vi "Main.vi"(11 "Module Admin":refnum<class "Delacor_lib_QMH_Module Admin.lvclass">) -> ()   [LabVIEW 2020, in "UI.lvlib"]
doc: "This template is based off of the Queued Message Handler design pattern and the Queued Message Handler project template that ships with LabVIEW.\n\nThe main difference is that the queue is private to this module and communication between modules is performed via Broadcast and Request events.\n\nRequest events are wrapped in public API methods and are handled in the Event Handling Loop (EHL) of this VI. Any module can register for Broadcast events sent by this module. The EHL generates messages based on user interface actions.\n\nThe Message Handling Loop (MHL) processes messages generated by the EHL, or by other messages. The messages are string values, so new messages can be added easily to the Message Cases case structure in the MHL. Each message cluster can also provide an optional value for Message Data, which is a variant that can be converted to whatever message-specific data is required.\n_____\nBased on DQMH Project Template 6.0.0.91."
uses:
  UI.lvlib
  <vilib>/Delacor/Delacor QMH/Libraries/Module Admin_class/Delacor_lib_QMH_Module Admin.lvclass
  Module Data--cluster.ctl
  Stop Argument--cluster.ctl
  <vilib>/Delacor/Delacor QMH/Libraries/Message Queue_class/Delacor_lib_QMH_Message Queue.lvclass/Delacor_lib_QMH_Message Queue.ctl
  <vilib>/Delacor/Delacor QMH/Libraries/Module Admin_class/Delacor_lib_QMH_Module Admin.lvclass/Delacor_lib_QMH_Module Admin.ctl
  <vilib>/Utility/miscctls.llb/LVPointTypeDef.ctl
  <vilib>/Delacor/Delacor QMH/Libraries/Message Queue_class/Delacor_lib_QMH_Enqueue Message (Single).vi
  <vilib>/Delacor/Delacor QMH/Libraries/Module Admin_class/Delacor_lib_QMH_Get External Launch.vi
  <vilib>/Utility/error.llb/Error Cluster From Error Code.vi
  <vilib>/ErrorRing/Error Ring.xnode
  <vilib>/Delacor/Delacor QMH/Libraries/Message Queue_class/Delacor_lib_QMH_Message Queue.lvclass
  Dinero/Dinero.lvlib
  Manejador Turnos/Manejador Turnos.lvlib
  Paquetes Disponibles/Paquetes Disponibles.lvlib
  Contabilidad/Contabilidad.lvlib
panel:
  in  "PARO TOTAL":bool
  in  "PARO":bool
  in  "Contabilidad":bool
  out "Status":string
  out "error out":errorcluster
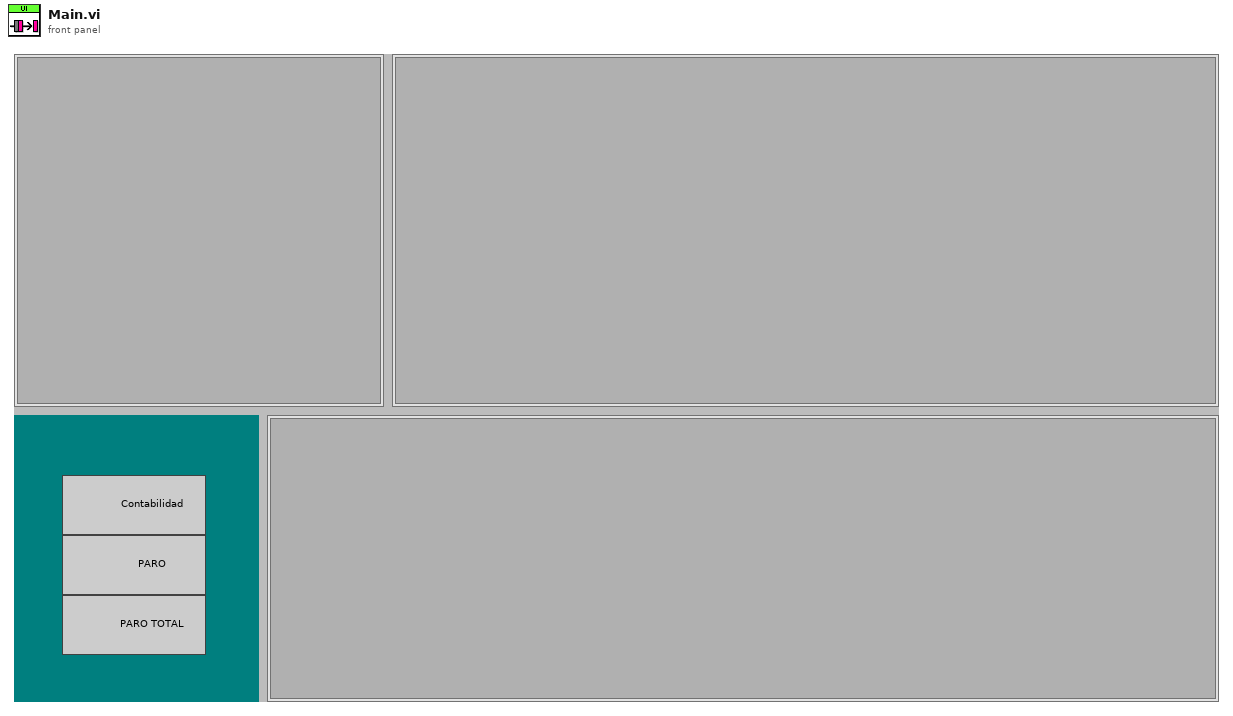
[diagram p1: front panel]
types:
  T1 = typedef "UI.lvlib/Request Events--cluster.ctl" = cluster{"Stop Module":refnum<user-event>, "Show Panel":refnum<user-event>, "Hide Panel":refnum<user-event>, "Get Module Execution Status":refnum<user-event>, "Show Diagram":refnum<user-event>, "Actualizar Cambio":refnum<user-event>, "Credito 0":refnum<user-event>}
  T2 = typedef "Contabilidad.lvlib/Broadcast Events--cluster.ctl" = cluster{"Module Did Init":refnum<user-event>, "Status Updated":refnum<user-event>, "Error Reported":refnum<user-event>, "Module Did Stop":refnum<user-event>, "Update Module Execution Status":refnum<user-event>}
  T3 = typedef "Manejador Turnos.lvlib/Broadcast Events--cluster.ctl" = cluster{"Module Did Init":refnum<user-event>, "Status Updated":refnum<user-event>, "Error Reported":refnum<user-event>, "Module Did Stop":refnum<user-event>, "Update Module Execution Status":refnum<user-event>}
  T4 = typedef "Paquetes Disponibles.lvlib/Broadcast Events--cluster.ctl" = cluster{"Module Did Init":refnum<user-event>, "Status Updated":refnum<user-event>, "Error Reported":refnum<user-event>, "Module Did Stop":refnum<user-event>, "Update Module Execution Status":refnum<user-event>, "Servicio Seleccionado":refnum<user-event>, "Actualizar Credito":refnum<user-event>, "Actualizar Cambio":refnum<user-event>}
  T5 = typedef "Dinero.lvlib/Broadcast Events--cluster.ctl" = cluster{"Module Did Init":refnum<user-event>, "Status Updated":refnum<user-event>, "Error Reported":refnum<user-event>, "Module Did Stop":refnum<user-event>, "Update Module Execution Status":refnum<user-event>, "Credito":refnum<user-event>}
  T6 = typedef "UI.lvlib/Module Data--cluster.ctl" = cluster{"Status":string}
  T7 = enum32{"invalid lock state", "Not Locked", "Locked (No Password)", "Password-protected"}
  T8 = typedef "UI.lvlib/Stop Argument--cluster.ctl" = cluster{"Origin":string, "Exit via Stop Module Req?":bool, "Wait for Module to stop?":bool}
  T9 = enum32{"Invalid", "Standard", "Closed", "Hidden", "Minimized", "Maximized"}
  T10 = typedef "LVPointTypeDef.ctl" = cluster{"Horizontal":i16, "Vertical":i16}
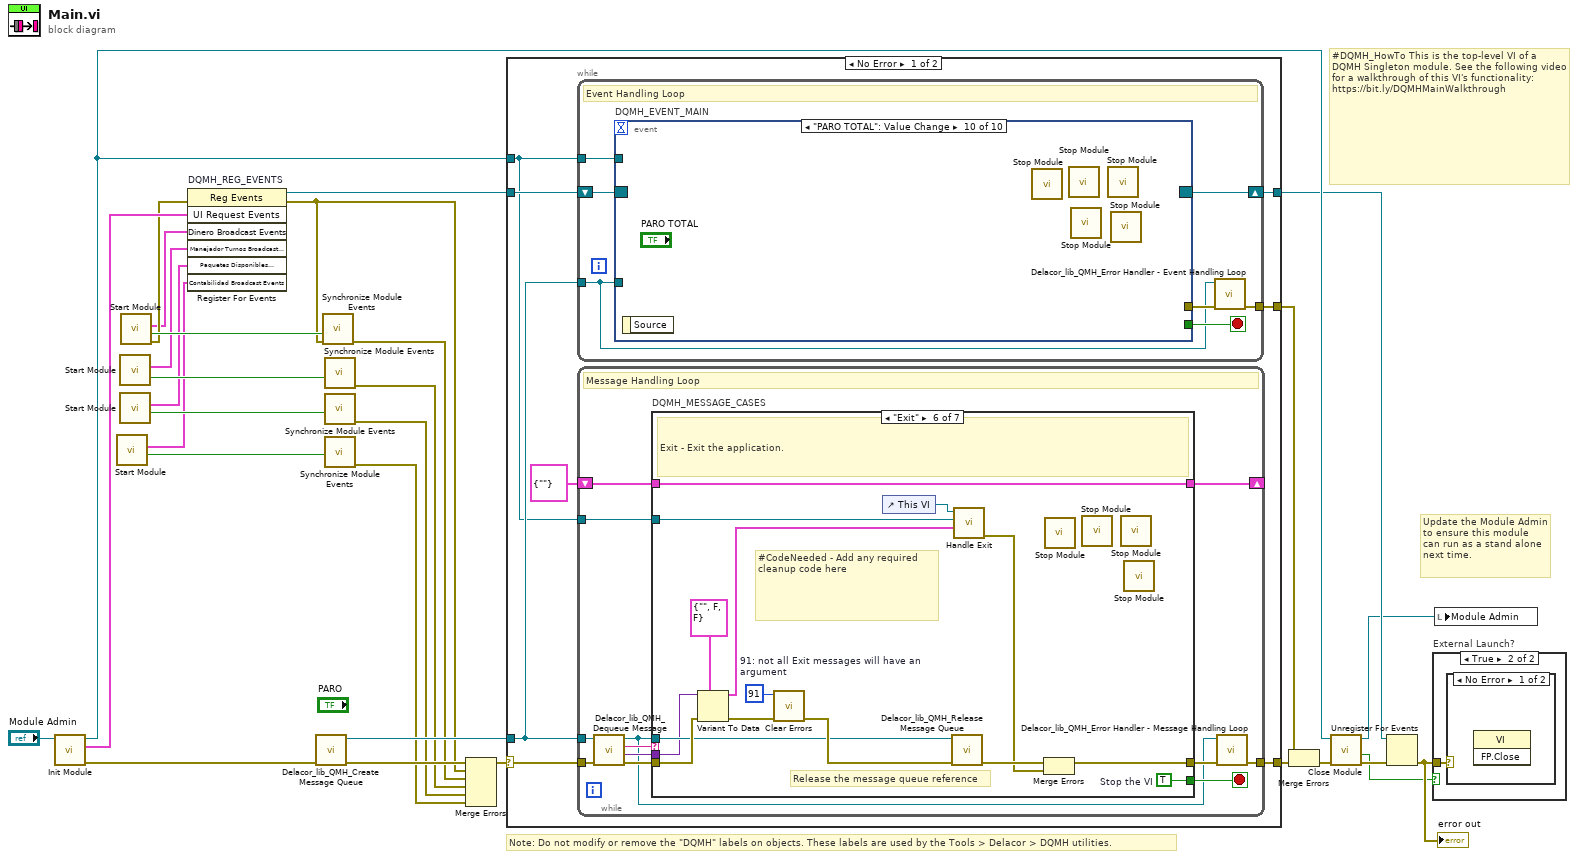
[diagram p0: block diagram]
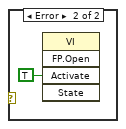
[diagram p3: hidden frame]
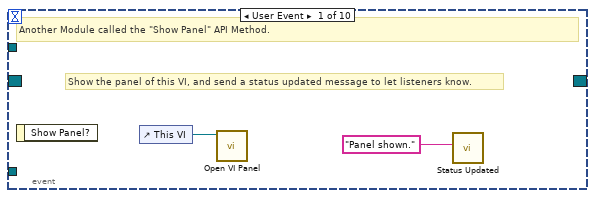
[diagram p4: hidden frame]
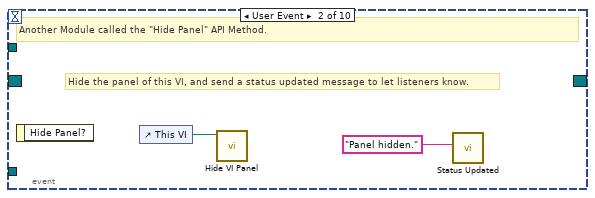
[diagram p5: hidden frame]
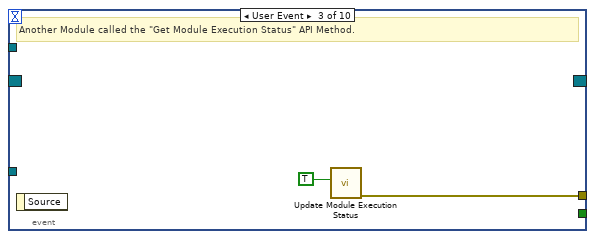
[diagram p6: hidden frame]
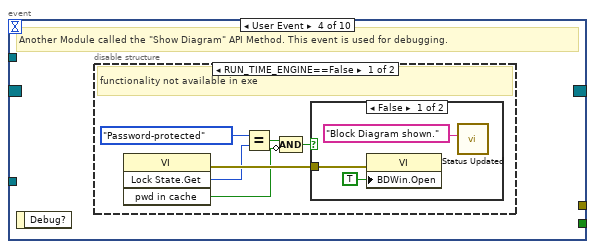
[diagram p7: hidden frame]
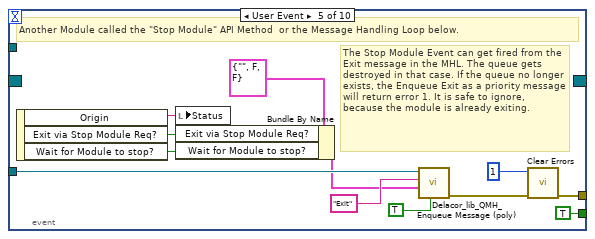
[diagram p10: hidden frame]
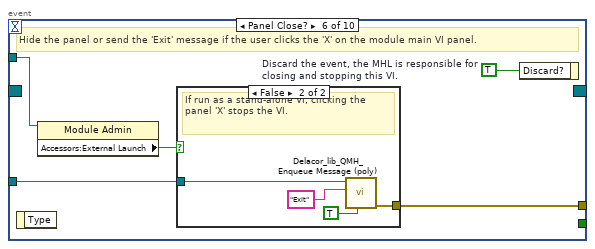
[diagram p11: hidden frame]
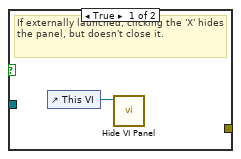
[diagram p12: hidden frame]
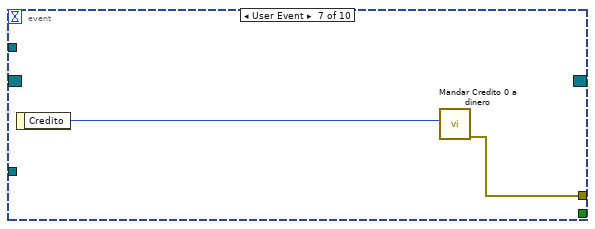
[diagram p13: hidden frame]
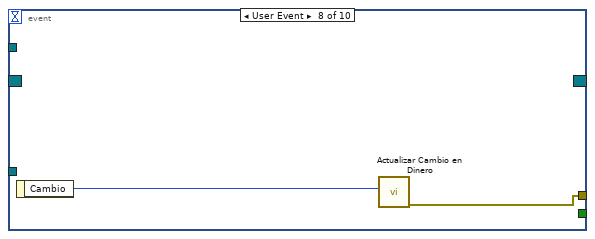
[diagram p14: hidden frame]
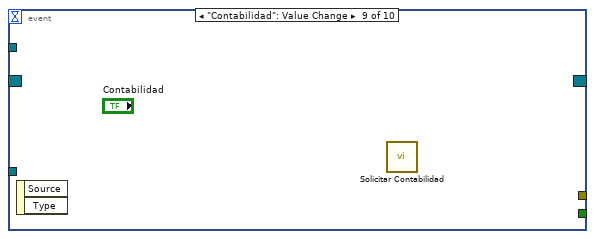
[diagram p15: hidden frame]
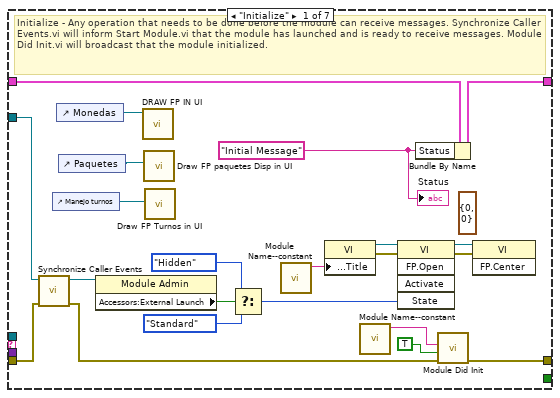
[diagram p16: hidden frame]
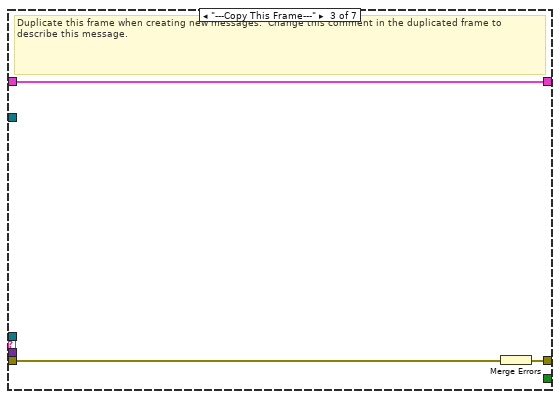
[diagram p18: hidden frame]
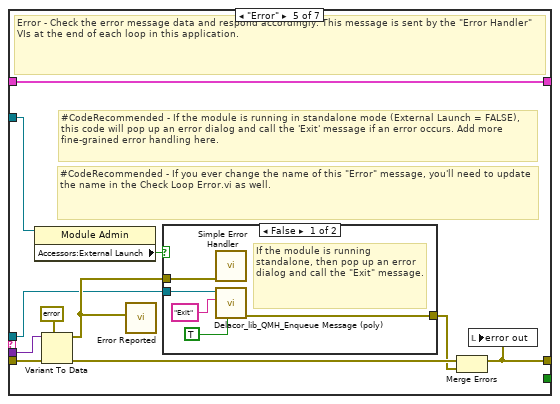
[diagram p20: hidden frame]
diagram:
  # "#DQMH_HowTo This is the top-level VI of a DQMH Singleton module. See the following video for a walkthrough of this VI's functionality: https://bit.ly/DQMHMainWalkthrough"
  # "Note: Do not modify or remove the \"DQMH\" labels on objects. These labels are used by the Tools > Delacor > DQMH utilities."
  # "Update the Module Admin to ensure this module can run as a stand alone next time."
  n1 = call "Init Module.vi"("Singleton Module Admin in"="Module Admin") -> ("error out"=w29:errorcluster, "UI Request Events"=w19:T1, "Singleton Module Admin out"=w22:refnum<class "Delacor_lib_QMH_Module Admin.lvclass">)  [unwired: 8 in]
  n2 = call "Start Module.vi"() -> ("Wait for Event Sync?"=w3:bool, "Contabilidad Broadcast Events"=w2:T2)  [unwired: 8 in, 2 out]
  n3 = call "Start Module.vi"() -> ("Wait for Event Sync?"=w9:bool, "Manejador Turnos Broadcast Events"=w5:T3)  [unwired: 8 in, 2 out]
  n4 = call "Start Module.vi"() -> ("Wait for Event Sync?"=w8:bool, "Paquetes Disponibles Broadcast Events"=w4:T4)  [unwired: 8 in, 2 out]
  n5 = call "Start Module.vi"() -> ("error out"=w13:errorcluster, "Wait for Event Sync?"=w14:bool, "Dinero Broadcast Events"=w10:T5)  [unwired: 8 in, 1 out]
  n6 = register-events "DQMH_REG_EVENTS"(error in=w13, w19, w10, w5, w4, w2) -> (reference out=w20:refnum<event-registration>, error out=w12:errorcluster)  [unwired: 1 in]
  n7 = call <vilib>:"Delacor_lib_QMH_Create Message Queue.vi"("error in"=w29) -> ("error out"=w24:errorcluster, "Message Queue"=w18:refnum<class "Delacor_lib_QMH_Message Queue.lvclass">)  [unwired: 9 in]
  n8 = call "Synchronize Module Events.vi"("error in"=w12, "Wait for Event Sync?"=w14) -> ("error out"=w11:errorcluster)  [unwired: 9 in]
  n9 = call "Synchronize Module Events.vi"("Wait for Event Sync?"=w9) -> ("error out"=w7:errorcluster)  [unwired: 10 in]
  n10 = call "Synchronize Module Events.vi"("Wait for Event Sync?"=w8) -> ("error out"=w6:errorcluster)  [unwired: 10 in]
  n11 = call "Synchronize Module Events.vi"("Wait for Event Sync?"=w3) -> ("error out"=w1:errorcluster)  [unwired: 10 in]
  n12 = Merge Errors(w24, w12, w11, w7, w6, w1) -> (w23:errorcluster)
  n13 = case shown="No Error" w23 {
    selector: w23 -> [w36 w175]
    tunnel: [w38 w174] -> w30
    tunnel: [w35 w180] -> w21
    tunnel: w20 -> [w33 w180]
    tunnel: w18 -> [w32 w173]
    tunnel: [w37 _] -> w27
    tunnel: w22 -> [w31 w176]
    frame No Error {
      n14 = while {
        tunnel: w32 -> [w39]
        shift-right: [w42] -> w35
        shift-left: w33 -> [w43]
        tunnel: [w44] -> w37
        tunnel: w31 -> [w40]
        stop <- w41 stop-if-true
        # "Event Handling Loop"
        n15 = event "DQMH_EVENT_MAIN" shown="[9] \"PARO TOTAL\": Value Change" {
          selector: w43 -> [_ _ _ _ _ _ _ _ _ _]
          dyn-events: [_ _ _ _ _ _ _ _ _ _] -> w42
          timeout: _ -> [_ _ _ _ _ _ _ _ _ _]
          tunnel: [_ _ _ _ TRUE ("Discard?") _ _ _ _ _] -> w41
          tunnel: w39 -> [_ _ _ _ w68 w75 _ _ _ _]
          tunnel: [_ _ w51 _ w71 w77 w83 w86 _ _] -> w45
          tunnel: w40 -> [_ _ _ _ _ w74 _ _ _ _]
          event User Event {
            # "Show the panel of this VI, and send a status updated message to let listeners know."
            # "Another Module called the \"Show Panel\" API Method."
            n16 = event-data() -> ()  [unwired: 1 in, 1 out]
            n17 = control-ref of="This VI"() -> (w47:refnum<vi>)
            n18 = call "Open VI Panel.vi"("VI"=w47) -> ()  [unwired: 10 in, 1 out]
            n19 = call "Status Updated.vi"("Status"="Panel shown." ("format string")) -> ()  [unwired: 10 in, 1 out]
          }
          event User Event {
            # "Hide the panel of this VI, and send a status updated message to let listeners know."
            # "Another Module called the \"Hide Panel\" API Method."
            n20 = event-data() -> ()  [unwired: 1 in, 1 out]
            n21 = control-ref of="This VI"() -> (w49:refnum<vi>)
            n22 = call "Hide VI Panel.vi"("VI"=w49) -> ()  [unwired: 10 in, 1 out]
            n23 = call "Status Updated.vi"("Status"="Panel hidden." ("format string")) -> ()  [unwired: 10 in, 1 out]
          }
          event User Event {
            # "Another Module called the \"Get Module Execution Status\" API Method."
            n24 = event-data() -> ()  [unwired: 1 in, 1 out]
            n25 = call "Update Module Execution Status.vi"("Running?"=TRUE) -> ("error out"=w51:errorcluster)  [unwired: 10 in]
          }
          event User Event {
            # "Another Module called the \"Show Diagram\" API Method. This event is used for debugging."
            n26 = event-data() -> ()  [unwired: 1 in, 1 out]
            n27 = disable-structure shown="RUN_TIME_ENGINE==False" {
              frame condition #0 (active) {
                # "functionality not available in exe"
                n28 = invoke class="VI" method="Lock State.Get"() -> (error out=w57:errorcluster, "Get Lock State"=w56:T7, "pwd in cache"=w53:bool)  [unwired: 4 in, 1 out]
                n29 = Equal?(x=T7."Password-protected", y=w56) -> (x = y?=w54:bool)
                n30 = Compound Arithmetic op=AND(w54, invert w53) -> (w52:bool)
                n31 = case shown="False" w52 {
                  tunnel: w57 -> [w60 _]
                  frame False {
                    n32 = property class="VI"(error in=w60, "BDWin.Open"=TRUE ("Block Diagram Window:Open")) -> ()  [unwired: 1 in, 2 out]
                    n33 = call "Status Updated.vi"("Status"="Block Diagram shown." ("format string")) -> ()  [unwired: 10 in, 1 out]
                  }
                  frame True {
                    # "Password-protected VI, and the password is not in the cache. Do not show the diagram."
                  }
                }
              }
              frame condition #1 {
              }
            }
          }
          event User Event {
            # "The Stop Module Event can get fired from the Exit message in the MHL. The queue gets destroyed in that case. If the queue no longer exists, the Enqueue Exit as a priority message will return error 1. It is safe to ignore, because the module is already exiting."
            # "Another Module called the \"Stop Module\" API Method  or the Message Handling Loop below."
            n34 = event-data() -> ("Origin"=w67:string, "Exit via Stop Module Req?"=w63:bool, "Wait for Module to stop?"=w62:bool)  [unwired: 1 in]
            n35 = local write "Status"(w67) -> ()
            n36 = Bundle By Name(cluster=T8 {"Origin"="", "Exit via Stop Module Req?"=FALSE, "Wait for Module to stop?"=FALSE} ("Stop Argument"), "Exit via Stop Module Req?"=w63, "Wait for Module to stop?"=w62) -> (w61:T8)
            n37 = call-poly <vilib>:"Delacor_lib_QMH_Enqueue Message (poly).vi"("Priority Message? (F)"=TRUE, "Message Data"=w61, "Message"="Exit", "Message Queue in"=w68) -> ("error out"=w72:errorcluster)  [unwired: 6 in, 1 out]
            n38 = call <vilib>:"Clear Errors.vi"("error in (no error)"=w72, "specific error code to clear (0: all)"=1) -> ("error out"=w71:errorcluster)  [unwired: 4 in, 1 out]
          }
          event Panel Close? {
            w76 = TRUE  # Discard the event, the MHL is responsible for closing and stopping this VI.
            # "Hide the panel or send the 'Exit' message if the user clicks the 'X' on the module main VI panel."
            n39 = event-data() -> ()  [unwired: 1 in, 1 out]
            n40 = property class="Module Admin"(reference=w74) -> ("Accessors:External Launch"=w73:bool)  [unwired: 1 in, 2 out]
            n41 = case shown="False" w73 {
              tunnel: w75 -> [_ w81]
              tunnel: [_ w82] -> w77
              frame True {
                # "If externally launched, clicking the 'X' hides the panel, but doesn't close it."
                n42 = control-ref of="This VI"() -> (w78:refnum<vi>)
                n43 = call "Hide VI Panel.vi"("VI"=w78) -> ()  [unwired: 10 in, 1 out]
              }
              frame False {
                # "If run as a stand-alone VI, clicking the panel 'X' stops the VI."
                n44 = call-poly <vilib>:"Delacor_lib_QMH_Enqueue Message (poly).vi"("Priority Message? (F)"=TRUE, "Message"="Exit", "Message Queue in"=w81) -> ("error out"=w82:errorcluster)  [unwired: 7 in, 1 out]
              }
            }
            n45 = event-data("Discard?"=w76) -> ()  [unwired: 1 in, 1 out]
          }
          event User Event {
            n46 = event-data() -> ("Credito"=w84:i32)  [unwired: 1 in]
            n47 = call "Mandar Credito 0 a dinero.vi"("Credito"=w84) -> ("error out"=w83:errorcluster)  [unwired: 10 in]
          }
          event User Event {
            n48 = event-data() -> ("Cambio"=w85:i32)  [unwired: 1 in]
            n49 = call "Actualizar Cambio en Dinero.vi"("Cambio"=w85) -> ("error out"=w86:errorcluster)  [unwired: 10 in]
          }
          event "Contabilidad": Value Change {
            n50 = event-data() -> ()  [unwired: 1 in, 2 out]
            n51 = call "Solicitar Contabilidad.vi"() -> ()  [unwired: 12 in]
          }
          event "PARO TOTAL": Value Change {
            n52 = event-data() -> ()  [unwired: 1 in, 1 out]
            n53 = call "Stop Module.vi"() -> ()  [unwired: 11 in, 1 out]
            n54 = call "Stop Module.vi"() -> ()  [unwired: 11 in, 1 out]
            n55 = call "Stop Module.vi"() -> ()  [unwired: 11 in, 1 out]
            n56 = call "Stop Module.vi"() -> ()  [unwired: 11 in, 1 out]
            n57 = call "Stop Module.vi"() -> ()  [unwired: 11 in, 1 out]
          }
        }
        n58 = call-dynamic "Delacor_lib_QMH_Error Handler - Event Handling Loop.vi"("error in"=w45, "Message Queue in"=w39) -> ("dup error in"=w44:errorcluster)  [unwired: 8 in, 1 out]
      }
      n59 = while {
        tunnel: w32 -> [w89]
        shift-right: [w93] -> _
        shift-left: T6 {"Status"=""} ("Data Cluster") -> [w94]
        tunnel: w36 -> [w97]
        tunnel: [w95] -> w38
        tunnel: w31 -> [w87]
        stop <- w92 stop-if-true
        # "Message Handling Loop"
        n60 = call-dynamic "Delacor_lib_QMH_Dequeue Message.vi"("error in"=w97, "Message Queue in"=w89) -> ("error out"=w96:errorcluster, "Message Data"=w90:variant, "Message"=w91:string, "Message Queue out"=w88:refnum<class "Delacor_lib_QMH_Message Queue.lvclass">)  [unwired: 6 in]
        n61 = case "DQMH_MESSAGE_CASES" shown="\"Exit\"" w91 {
          selector: w91 -> [_ _ _ _ _ _ w160]
          tunnel: w88 -> [_ _ _ _ w130 w152 _]
          tunnel: w96 -> [w118 w122 w125 w127 w137 w158 w162]
          tunnel: [w116 w122 w124 w127 w133 w155 w163] -> w98
          tunnel: w94 -> [w107 w121 w123 w126 w132 w151 w161]
          tunnel: [w106 w121 w123 w126 w132 w151 w161] -> w93
          tunnel: [_ _ _ _ _ w150 _] -> w92
          tunnel: w90 -> [_ _ _ _ w131 w149 _]
          tunnel: w87 -> [w108 _ _ _ w129 w144 _]
          frame "Initialize" {
            (unwired) T10 {"Horizontal"=0, "Vertical"=0} ("Origin")
            w102 = "Initial Message" ("Initial Message")
            # "Initialize - Any operation that needs to be done before the module can receive messages. Synchronize Caller Events.vi will inform Start Module.vi that the module has launched and is ready to receive messages. Module Did Init.vi will broadcast that the module initialized."
            n62 = call "Synchronize Caller Events.vi"("error in (no error)"=w118, "Singleton Module Admin in"=w108) -> ("error out"=w117:errorcluster, "Singleton Module Admin out"=w103:refnum<class "Delacor_lib_QMH_Module Admin.lvclass">)  [unwired: 8 in]
            n63 = control-ref of="Manejo turnos"() -> (w99:refnum<vi>)
            n64 = control-ref of="Monedas"() -> (w101:refnum<vi>)
            n65 = control-ref of="Paquetes"() -> (w100:refnum<vi>)
            n66 = property class="Module Admin"(reference=w103) -> ("Accessors:External Launch"=w112:bool)  [unwired: 1 in, 2 out]
            n67 = call "DRAW FP IN UI.vi"("Sub Panel Dinero"=w101) -> ()  [unwired: 10 in, 1 out]
            n68 = call "Draw FP paquetes Disp in UI.vi"("Sub Panel Paquetes"=w100) -> ()  [unwired: 10 in, 1 out]
            n69 = call "Draw FP Turnos in UI.vi"("Sub Panel Trunos"=w99) -> ()  [unwired: 10 in, 1 out]
            n70 = Select(t=T9."Hidden" ("State"), s=w112, f=T9."Standard" ("State")) -> (s? t:f=w109:T9)
            n71 = call "Module Name--constant.vi"() -> ("Module Name"=w115:string)  [unwired: 11 in]
            n72 = property class="VI"("Front Panel.Title"=w115) -> (reference out=w114:refnum<vi>, error out=w120:errorcluster)  [unwired: 2 in]
            n73 = call "Module Name--constant.vi"() -> ("Module Name"=w104:string)  [unwired: 11 in]
            n74 = invoke class="VI" method="FP.Open"(reference=w114, error in=w120, "State"=w109) -> (reference out=w113:refnum<vi>, error out=w119:errorcluster)  [unwired: 2 in, 3 out]
            n75 = Bundle By Name(cluster=w107, "Status"=w102) -> (w106:T6)
            n76 = call "Module Did Init.vi"("error in (no error)"=w117, "Initialized?"=TRUE, "Origin"=w104) -> ("error out"=w116:errorcluster)  [unwired: 8 in]
            n77 = invoke class="VI" method="FP.Center"(reference=w113, error in=w119) -> ()  [unwired: 1 in, 3 out]
            "Status" <- w102
          }
          frame "---Module Specific---" {
            # "Separator -- The following cases handle messages specific to this Module."
          }
          frame "---Copy This Frame---" {
            # "Duplicate this frame when creating new messages.  Change this comment in the duplicated frame to describe this message."
            n78 = Merge Errors(w125) -> (w124:errorcluster)
          }
          frame "---Exit and Error Handling---" {
            # "Separator - The following cases handle errors and exit messages."
          }
          frame "Error" {
            # "#CodeRecommended - If you ever change the name of this \"Error\" message, you'll need to update the name in the Check Loop Error.vi as well."
            # "#CodeRecommended - If the module is running in standalone mode (External Launch = FALSE), this code will pop up an error dialog and call the 'Exit' message if an error occurs. Add more fine-grained error handling here."
            # "Error - Check the error message data and respond accordingly. This message is sent by the \"Error Handler\" VIs at the end of each loop in this application."
            n79 = property class="Module Admin"(reference=w129) -> ("Accessors:External Launch"=w128:bool)  [unwired: 1 in, 2 out]
            n80 = Variant To Data(error in=w137, type=errorcluster {"status"=FALSE, "code"=0, "source"=""} ("error constant"), Variant=w131) -> (data=w138:errorcluster, error out=w135:errorcluster)
            n81 = call "Error Reported.vi"("Error"=w138) -> ()  [unwired: 10 in, 1 out]
            n82 = case shown="False" w128 {
              tunnel: [w143 _] -> w134
              tunnel: w130 -> [w141 _]
              tunnel: w138 -> [w142 _]
              frame False {
                # "If the module is running standalone, then pop up an error dialog and call the \"Exit\" message."
                n83 = call <vilib>:"Simple Error Handler.vi"("error in (no error)"=w142) -> ()  [unwired: 4 in, 5 out]
                n84 = call-poly <vilib>:"Delacor_lib_QMH_Enqueue Message (poly).vi"("Priority Message? (F)"=TRUE, "Message"="Exit", "Message Queue in"=w141) -> ("error out"=w143:errorcluster)  [unwired: 7 in, 1 out]
              }
              frame True {
                # "If the module was launched externally, calling the Error Reported broadcast VI is the only action performed by the \"Error\" message. The module's caller can then process the error appropriately."
              }
            }
            n85 = Merge Errors(w135, w134) -> (w133:errorcluster)
            n86 = local write "error out"(w133) -> ()
          }
          frame "Exit" {
            w148 = 91  # 91: not all Exit messages will have an argument
            w150 = TRUE  # Stop the VI
            # "Release the message queue reference"
            # "#CodeNeeded - Add any required cleanup code here"
            # "Exit - Exit the application."
            n87 = Variant To Data(error in=w158, type=T8 {"Origin"="", "Exit via Stop Module Req?"=FALSE, "Wait for Module to stop?"=FALSE} ("Stop Argument"), Variant=w149) -> (data=w146:T8, error out=w154:errorcluster)
            n88 = call <vilib>:"Clear Errors.vi"("error in (no error)"=w154, "specific error code to clear (0: all)"=w148) -> ("error out"=w157:errorcluster)  [unwired: 4 in, 1 out]
            n89 = control-ref of="This VI"() -> (w145:refnum<vi>)
            n90 = call-dynamic "Delacor_lib_QMH_Release Message Queue.vi"("error in"=w157, "Message Queue"=w152) -> ("error out"=w156:errorcluster)  [unwired: 9 in]
            n91 = call "Handle Exit.vi"("Stop Argument"=w146, "Admin in"=w144, "VI reference"=w145) -> ("error out"=w153:errorcluster)  [unwired: 7 in, 1 out]
            n92 = Merge Errors(w156, w153) -> (w155:errorcluster)
            n93 = call "Stop Module.vi"() -> ()  [unwired: 11 in, 1 out]
            n94 = call "Stop Module.vi"() -> ()  [unwired: 11 in, 1 out]
            n95 = call "Stop Module.vi"() -> ()  [unwired: 11 in, 1 out]
            n96 = call "Stop Module.vi"() -> ()  [unwired: 11 in, 1 out]
          }
          frame Default {
            # "'Default' case only runs if there is a message that isn't defined in any of the other cases.  Output a programming error."
            n97 = call "Module Name--constant.vi"() -> ("Module Name"=w159:string)  [unwired: 11 in]
            n98 = xnode "Error Ring"("parameter 0"=w160, "parameter 1"=w159) -> ("error out"=w164:errorcluster)
            n99 = Merge Errors(w162, w164) -> (w163:errorcluster)
          }
        }
        n100 = call-dynamic "Delacor_lib_QMH_Error Handler - Message Handling Loop.vi"("error in"=w98, "Message Queue in"=w88) -> ("dup error in"=w95:errorcluster)  [unwired: 8 in, 1 out]
      }
    }
    frame Error {
      # "Synchronize Caller Events.vi will inform Start Module.vi that the module has launched and will let the code calling Start Module.vi register for broadcasts and would permit the caller receive the broadcast that an error occurred at launch time."
      n101 = call-dynamic "Delacor_lib_QMH_Release Message Queue.vi"("error in"=w175, "Message Queue"=w173) -> ("error out"=w174:errorcluster)  [unwired: 9 in]
      n102 = call "Synchronize Caller Events.vi"("Singleton Module Admin in"=w176) -> ("error out"=w181:errorcluster)  [unwired: 9 in, 1 out]
      n103 = call "Module Name--constant.vi"() -> ("Module Name"=w179:string)  [unwired: 11 in]
      n104 = Format Into String(format string="An error occurred during initialization. %s is no longer running.", w179) -> (resulting string=w177:string)  [unwired: 2 in, 1 out]
      n105 = Merge Errors(w174, w181) -> (w182:errorcluster)
      n106 = call "Error Reported.vi"("Additional Information"=w177, "Error"=w182) -> ()  [unwired: 9 in, 1 out]
      n107 = call "Stop Module.vi"() -> ()  [unwired: 11 in, 1 out]
      n108 = call "Stop Module.vi"() -> ()  [unwired: 11 in, 1 out]
      n109 = call "Stop Module.vi"() -> ()  [unwired: 11 in, 1 out]
      n110 = call "Stop Module.vi"() -> ()  [unwired: 11 in, 1 out]
    }
  }
  n111 = Merge Errors(w27, w30) -> (w26:errorcluster)
  n112 = call "Close Module.vi"("error in (no error)"=w26, "Module Admin in"=w22) -> ("error out"=w28:errorcluster, "External Launch"=w15:bool, "Module Admin out"=w16:refnum<class "Delacor_lib_QMH_Module Admin.lvclass">)  [unwired: 7 in]
  n113 = Unregister For Events(event registration refnum=w21, error in=w28) -> (error out=w25:errorcluster)
  "error out" <- w25
  n114 = case "External Launch?" shown="True" w15 {
    tunnel: w25 -> [_ w183]
    frame False {
    }
    frame True {
      n115 = case shown="No Error" w183 {
        frame No Error {
          n116 = invoke class="VI" method="FP.Close"() -> ()  [unwired: 3 in, 3 out]
        }
        frame Error {
          n117 = invoke class="VI" method="FP.Open"("Activate"=TRUE ("Activate?")) -> ()  [unwired: 4 in, 5 out]
        }
      }
    }
  }
  n118 = local write "Module Admin"(w16) -> ()
